vi "Get JSON Example.vi"(6 "type":enum16{"request", "response"}(ring), 8 "error in (no error)":errorcluster, 9 "params or result":variant, 10 "method":string) -> (0 "error out":errorcluster, 2 "<JSON>":string)   [LabVIEW 2019, in "Help.lvclass"]
doc: "Given a <b>method</b> name and <b>params</b> (if a request) or <b>result</b> (if a response) cluster this VI will return an example jsonrpc object"
uses:
  Help.lvclass
  <userlib>/LevyLab/JSON-RPC/JSON-RPC.lvlib
  <vilib>/Utility/Data Type/NI_Data Type.lvlib
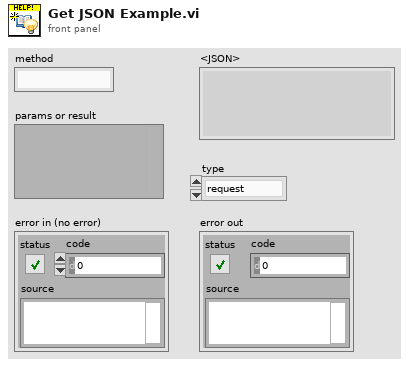
[diagram p1: front panel]
types:
  T1 = typedef "NI_Data Type.lvlib/Data Type.ctl" = enum8{"Invalid Type", "Void", "I8", "I16", "I32", "I64", "U8", "U16", "U32", "U64", "Single Float", "Double Float", "Extended Float", "Single Complex", "Double Complex", "Extended Complex", "Enum U8", "Enum U16", "Enum U32", "Enum U64", "Single Float With Unit", "Double Float With Unit", "Extended Float With Unit", "Single Complex with Unit", "Double Complex with Unit", "Extended Complex with Unit", "Boolean", "String", "Path", "Picture", "Tag", "Array", "Cluster", "Variant", "LV Variant", "Waveform", "Timestamp", "Digital Waveform", "Digital Data", "ExpressData", "Refnum", "External Data", "VI", "Poly VI", "LabVIEW Class Instance", "Fixed Point", "Set Collection", "Map Collection"}
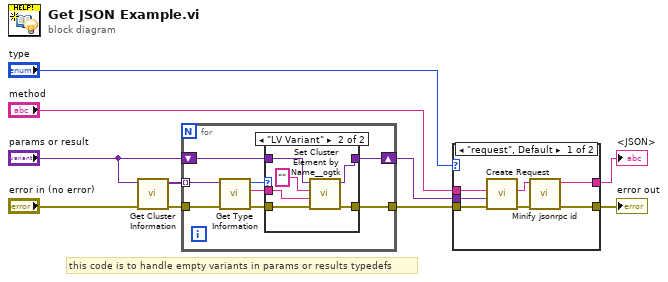
[diagram p0: block diagram]
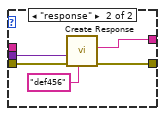
[diagram p2: hidden frame]
diagram:
  # "this code is to handle empty variants in params or results typedefs"
  n1 = call <vilib>:"Get Cluster Information.vi"("error in (no error)"="error in (no error)", "variant"="params or result") -> ("error out"=w6:errorcluster, "cluster elements"=w7:variant[])  [unwired: 8 in]
  n2 = for {
    shift-right: [w14] -> w4
    shift-left: "params or result" -> [w15]
    tunnel: w7 -> [w18] mode=indexing
    tunnel: w6 -> [w17]
    tunnel: [w12] -> w3
    n3 = call <vilib>:"Get Type Information.vi"("error in (no error)"=w17, "variant"=w18) -> ("error out"=w13:errorcluster, "name"=w11:string, "type"=w16:T1)  [unwired: 5 in, 2 out]
    n4 = case shown="\"LV Variant\"" w16 {
      tunnel: w15 -> [w20 w25]
      tunnel: [w20 w24] -> w14
      tunnel: w13 -> [w19 w21]
      tunnel: [w19 w26] -> w12
      tunnel: w11 -> [_ w23]
      frame Default {
      }
      frame "LV Variant" {
        n5 = call <userlib>:"Set Cluster Element by Name__ogtk.vi"("error in (no error)"=w21, "Element Name (\"\": New Element Data Name)"=w23, "New Element Value"="", "Cluster"=w25) -> ("error out"=w26:errorcluster, "VCluster out"=w24:variant)  [unwired: 5 in, 1 out]
      }
    }
  }
  n6 = case shown="\"request\", Default" "type" {
    tunnel: [w33 w35] -> w10
    tunnel: w3 -> [w32 w38]
    tunnel: "method" -> [w30 _]
    tunnel: w4 -> [w29 w37]
    tunnel: [w28 w34] -> w9
    frame "request", Default {
      n7 = call <userlib>:"Create Request.vi"("error in (no error)"=w32, "params"=w29, "method"=w30) -> ("error out"=w31:errorcluster, "<JSON> Requests"=w27:string)  [unwired: 6 in, 1 out]
      n8 = call "Minify jsonrpc id.vi"("error in (no error)"=w31, "<JSON> Requests"=w27) -> ("error out"=w33:errorcluster, "<JSON>"=w28:string)  [unwired: 8 in]
    }
    frame "response" {
      n9 = call <userlib>:"Create Response.vi"("id"="def456", "error in (no error)"=w38, "result"=w37) -> ("error out"=w35:errorcluster, "<JSON> Response"=w34:string)  [unwired: 7 in]
    }
  }
  "error out" <- w10
  "<JSON>" <- w9
